vi "Feature Vector.vi"(6 "Basis":enum16{"Polynomial", "Fourier"}(ring), 8 "n":i32=1, 11 "input":dbl[](array[numeric])=[0.1, 0.2, 0.3]) -> (3 "feature vector":dbl[](array[numeric])=[1.0, 0.1, 0.2, 0.020000000000000004, 0.3, 0.03, 0.06, 0.006000000000000001])   [LabVIEW 2017]
uses:
  <vilib>/Analysis/baseanly.llb/Real Dot Product.vi
  <vilib>/Analysis/NI_AALBase.lvlib
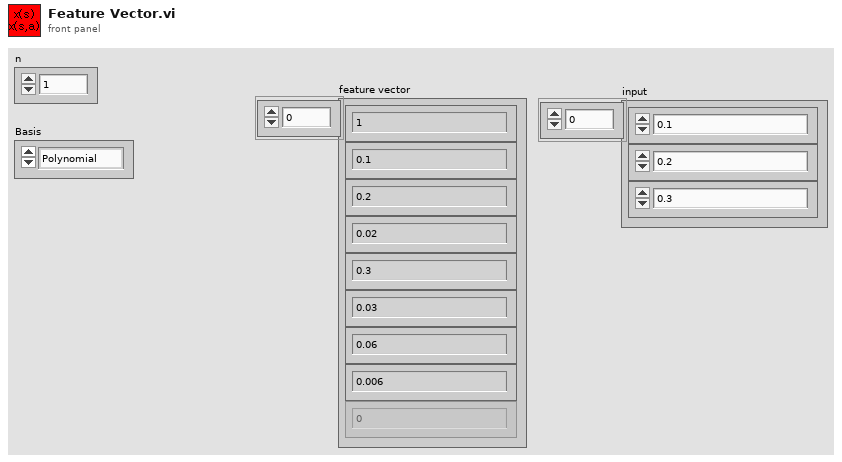
[diagram p1: front panel]
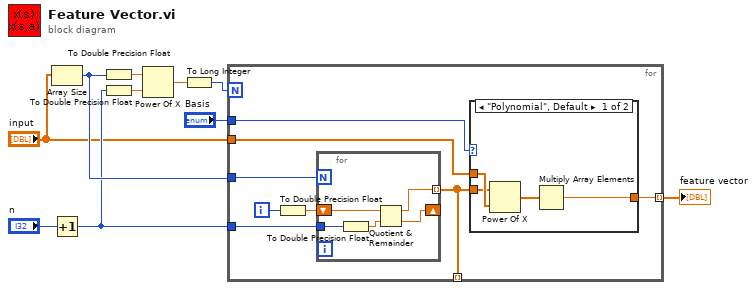
[diagram p0: block diagram]
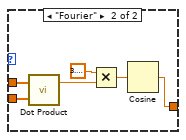
[diagram p2: hidden frame]
diagram:
  n1 = Array Size(array="input") -> (size(s)=w5:i32)
  n2 = Increment(x="n") -> (x+1=w4:i32)
  n3 = To Double Precision Float(number=w5) -> (double precision float=w8:dbl)
  n4 = To Double Precision Float(number=w4) -> (double precision float=w9:dbl)
  n5 = Power Of X(1:w9, 2:w8) -> (0:w7:dbl)
  n6 = To Long Integer(number=w7) -> (32bit integer=w6:i32)
  n7 = for {
    N: w6 -> [_]
    tunnel: w5 -> [w18]
    tunnel: w4 -> [w17]
    tunnel: "input" -> [w16]
    tunnel: [w15] -> w3 mode=indexing
    tunnel: "Basis" -> [w12]
    tunnel: [w11] -> _ mode=indexing
    i -> [w14]
    n8 = To Double Precision Float(number=w14) -> (double precision float=w13:dbl)
    n9 = for {
      N: w18 -> [_]
      shift-right: [w30] -> _
      shift-left: w13 -> [w29]
      tunnel: w17 -> [w33]
      tunnel: [w31] -> w11 mode=indexing
      n10 = To Double Precision Float(number=w33) -> (double precision float=w32:dbl)
      n11 = Quotient & Remainder(x=w29, y=w32) -> (x-y*floor(x/y)=w31:dbl, floor(x/y)=w30:dbl)
    }
    n12 = case shown="\"Polynomial\", Default" w12 {
      tunnel: w16 -> [w22 w28]
      tunnel: [w20 w23] -> w15
      tunnel: w11 -> [w19 w27]
      frame "Polynomial", Default {
        n13 = Power Of X(1:w22, 2:w19) -> (0:w21:dbl[])
        n14 = Multiply Array Elements(1:w21) -> (0:w20:dbl)
      }
      frame "Fourier" {
        n15 = call-poly <vilib>:"Dot Product.vi"("Y Vector"=w27, "X Vector"=w28) -> ("X * Y"=w26:dbl)  [unwired: 1 out]
        n16 = Multiply(x=3.141592653589793, y=w26) -> (x*y=w24:dbl)
        n17 = Cosine(x=w24) -> (cos(x)=w23:dbl)
      }
    }
  }
  "feature vector" <- w3
